vi "Speed Limiter.vi"(7 "Limit":dbl=0.8 format="%#_13g", 11 "Motor Input":dbl) -> (3 "Output":dbl)   [LabVIEW 2017]
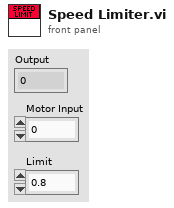
[diagram p1: front panel]
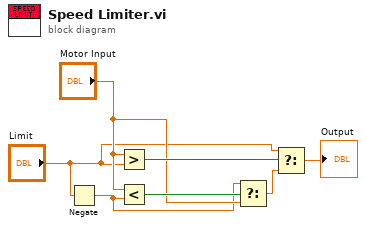
[diagram p0: block diagram]
diagram:
  n1 = Negate(x="Limit") -> (-x=w2:dbl)
  n2 = Greater?(x="Motor Input", y="Limit") -> (0:w7:bool)
  n3 = Less?(x="Motor Input", y=w2) -> (x < y?=w5:bool)
  n4 = Select(t=w2, s=w5, f="Motor Input") -> (s? t:f=w6:dbl)
  n5 = Select(t="Limit", s=w7, f=w6) -> (s? t:f=→"Output":dbl)
